vi "DistillTitle.vi"(7 "Plot Summary in":string[][](array[string]), 10 "Indices to include in Page Title":i32[](array[numeric]), 11 "String in":string) -> (3 "String out":string, 4 "AvailableVariables":string[](array[string]))   [LabVIEW 2012]
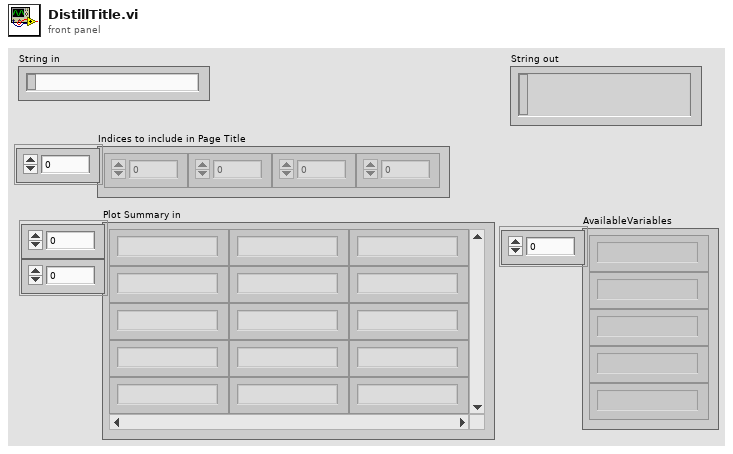
[diagram p1: front panel]
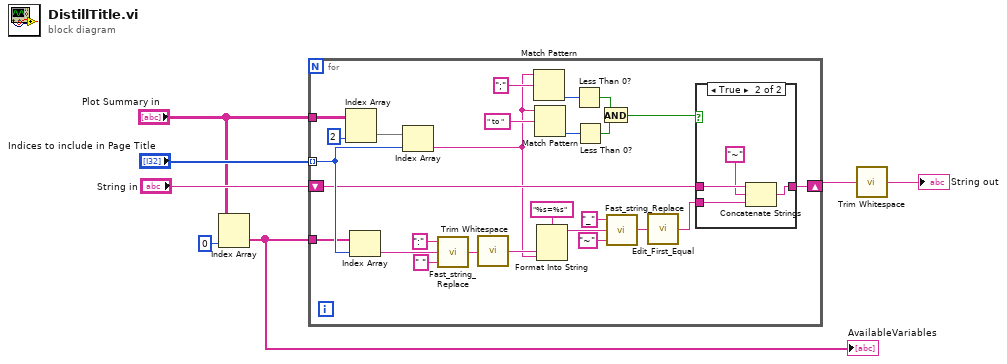
[diagram p0: block diagram]
diagram:
  n1 = Index Array(array="Plot Summary in", index (col)=0 ("disabled index (col)")) -> (element=w4:string[])  [unwired: 1 in]
  "AvailableVariables" <- w4
  n2 = for {
    tunnel: "Indices to include in Page Title" -> [w32] mode=indexing
    tunnel: "Plot Summary in" -> [w33]
    shift-right: [w23] -> w5
    shift-left: "String in" -> [w24]
    tunnel: w4 -> [w21]
    n3 = Index Array(array=w33, index (col)=2 ("index (row)")) -> (element=w31:string[])  [unwired: 1 in]
    n4 = Index Array(array=w21, index=w32) -> (element=w27:string)
    n5 = Index Array(array=w31, index=w32) -> (element=w18:string)
    n6 = call "Fast_string_Replace.vi"("Replace match with:"=" ", "Input String"=w27, "regular expression"=":") -> ("Output String"=w26:string)  [unwired: 2 out]
    n7 = call <vilib>:"Trim Whitespace.vi"("string"=w26) -> ("trimmed string"=w25:string)  [unwired: 1 in]
    n8 = Match Pattern(string=w18, regular expression=";") -> (offset past match=w14:i32)  [unwired: 4 out]
    n9 = Match Pattern(string=w18, regular expression=" to ") -> (offset past match=w15:i32)  [unwired: 4 out]
    n10 = Format Into String(format string="%s=%s", w25, w18) -> (resulting string=w10:string)  [unwired: 2 in, 1 out]
    n11 = Less Than 0?(x=w14) -> (x < 0?=w16:bool)
    n12 = Less Than 0?(x=w15) -> (x < 0?=w17:bool)
    n13 = And(x=w16, y=w17) -> (x .and. y?=w13:bool)
    n14 = call "Fast_string_Replace.vi"("Replace match with:"="~", "Input String"=w10, "regular expression"="_") -> ("Output String"=w9:string)  [unwired: 2 out]
    n15 = call "Edit_First_Equal.vi"("String in"=w9) -> ("String out"=w8:string)
    n16 = case shown="True" w13 {
      tunnel: w24 -> [w34 w38]
      tunnel: [w34 w37] -> w23
      tunnel: w8 -> [_ w36]
      frame False {
      }
      frame True {
        n17 = Concatenate Strings(w38, "~" ("string"), w36) -> (w37:string)
      }
    }
  }
  n18 = call <vilib>:"Trim Whitespace.vi"("string"=w5) -> ("trimmed string"=→"String out":string)  [unwired: 1 in]
